vi "Item Indent.vi"(0 "Tree Reference In":refnum<vi>, 2 "Indent Tag (Current)":string, 5 "error in (no error)":errorcluster) -> (14 "Tree Reference Out":refnum<vi>, 19 "error out":errorcluster)   [LabVIEW 2011, in "VITesterUtilities.lvlib"]
doc: "Takes the input tag item and places it along with its children as a child family of its current topmost sibling. Ignores the indent command if there is no current sibling to indent under."
uses:
  Libraries/VITesterUtilities.lvlib
panel:
  # "VI OUTPUTS"
  # "VI INPUTS"
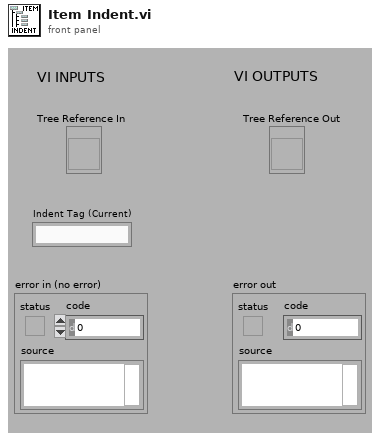
[diagram p1: front panel]
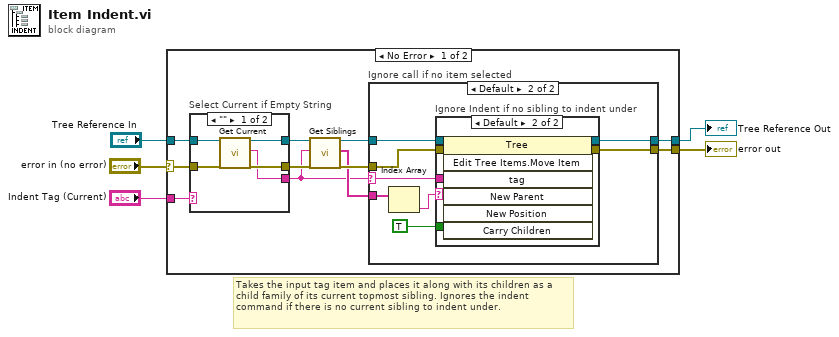
[diagram p0: block diagram]
diagram:
  # "Takes the input tag item and places it along with its children as a child family of its current topmost sibling. Ignores the indent command if there is no current sibling to indent under."
  n1 = case shown="No Error" "error in (no error)" {
    selector: "error in (no error)" -> [w14 w44]
    tunnel: "Tree Reference In" -> [w16 w45]
    tunnel: [w13 w45] -> w4
    tunnel: [w12 w44] -> w3
    tunnel: "Indent Tag (Current)" -> [w15 _]
    frame No Error {
      n2 = case "Select Current if Empty String" shown="\"\"" w15 {
        selector: w15 -> [_ w41]
        tunnel: [w39 w43] -> w11
        tunnel: w16 -> [w40 w43]
        tunnel: [w38 w42] -> w10
        tunnel: w14 -> [w37 w42]
        tunnel: [w36 w41] -> w6
        frame "" {
          n3 = call "Get Current.vi"("Tree Reference In"=w40, "error in (no error)"=w37) -> ("Tree Reference Out"=w39:refnum<vi>, "Current Tag"=w36:string, "error out"=w38:errorcluster)  [unwired: 14 in, 1 out]
        }
        frame Default {
        }
      }
      n4 = call "Get Siblings.vi"("Tree Reference In"=w11, "Input Tag (Current)"=w6, "error in (no error)"=w10) -> ("Tree Reference Out"=w9:refnum<vi>, "Sibling Tags"=w7:string[], "error out"=w8:errorcluster)  [unwired: 14 in]
      n5 = case "Ignore call if no item selected" shown="Default" w6 {
        selector: w6 -> [_ w19]
        tunnel: [w18 w26] -> w13
        tunnel: [w17 w25] -> w12
        tunnel: w9 -> [w18 w23]
        tunnel: w8 -> [w17 w22]
        tunnel: w7 -> [_ w21]
        frame "" {
        }
        frame Default {
          n6 = Index Array(array=w21) -> (element=w20:string)  [unwired: 1 in]
          n7 = case "Ignore Indent if no sibling to indent under" shown="Default" w20 {
            selector: w20 -> [_ w29]
            tunnel: [w28 w35] -> w26
            tunnel: [w27 w34] -> w25
            tunnel: TRUE ("Carry Children") -> [_ w33]
            tunnel: w23 -> [w28 w32]
            tunnel: w22 -> [w27 w31]
            tunnel: w19 -> [_ w30]
            frame "" {
            }
            frame Default {
              n8 = invoke class="Tree" method="Edit Tree Items.Move Item"(reference=w32, error in=w31, "tag"=w30, "New Parent"=w29, "Carry Children"=w33) -> (reference out=w35:refnum<vi>, error out=w34:errorcluster)  [unwired: 2 in, 5 out]
            }
          }
        }
      }
    }
    frame Error {
    }
  }
  "Tree Reference Out" <- w4
  "error out" <- w3
